vi "run-vi-test-fail.vi"(11 "args":string[](array[string])) -> (2 "error":string, 3 "code":i32)   [LabVIEW 2023]
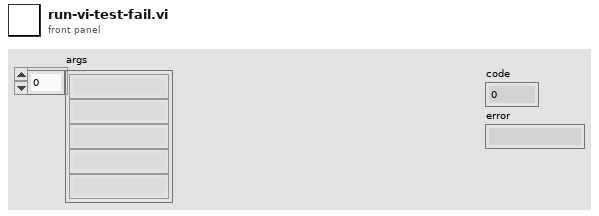
[diagram p1: front panel]
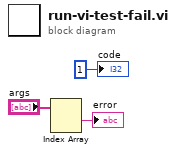
[diagram p0: block diagram]
diagram:
  n1 = Index Array(array="args") -> (element #1=→"error":string)  [unwired: 2 in, 1 out]
  "code" <- 1 ("code")
